vi "VariantToINIstring.vi"(7 "use system decimal point (T)":bool=TRUE, 11 "Variant-formatted Value":variant) -> (3 "String-formatted Value":string)   [LabVIEW 2013, in "OpenSerializer.lvlib" / "Serializer.PlainText.INI.lvclass"]
uses:
  Serializer.PlainText.INI.lvclass
  <vilib>/LabVIEW Open Source Project/Data Manipulation/TypeDescriptor/TypeDescriptor_GetName.vi
  <vilib>/LabVIEW Open Source Project/Data Manipulation/TypeDescriptor/TypeDescriptor_GetPString.vi
  <vilib>/LabVIEW Open Source Project/Data Manipulation/TypeDescriptor/TypeDescriptor_SetName.vi
  <vilib>/Utility/GetType.llb/Get Type Code from I16 Array And Pos.vi
  <vilib>/Utility/GetType.llb/TD_Get Array Information.vi
  <vilib>/LabVIEW Open Source Project/Data Manipulation/Conversions/Flattened nD-Array to Flattened 1D-Array.vi
  <vilib>/Utility/VariantDataType/VariantType.lvlib
  <vilib>/LabVIEW Open Source Project/Data Manipulation/Variant/OpenVariant.lvlib
  Serializer.PlainText/Serializer.PlainText.lvclass
  <vilib>/LabVIEW Open Source Project/Data Manipulation/TypeDescriptor/OpenDescriptor.lvlib
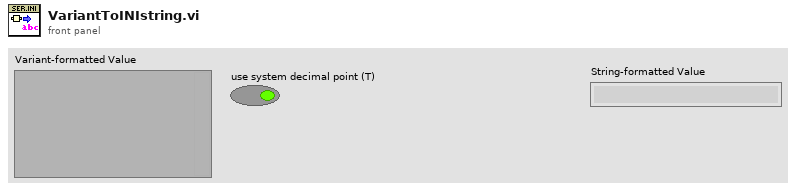
[diagram p1: front panel]
types:
  T1 = typedef "VariantType.lvlib/Type.ctl" = enum8{"Invalid Type", "Void", "I8", "I16", "I32", "I64", "U8", "U16", "U32", "U64", "Single Float", "Double Float", "Extended Float", "Single Complex", "Double Complex", "Extended Complex", "Enum U8", "Enum U16", "Enum U32", "Enum U64", "Single Float With Unit", "Double Float With Unit", "Extended Float With Unit", "Single Complex with Unit", "Double Complex with Unit", "Extended Complex with Unit", "Boolean", "String", "Path", "Picture", "Tag", "Array", "Cluster", "Variant", "LV Variant", "Waveform", "Timestamp", "Digital Waveform", "Digital Data", "ExpressData", "Refnum", "External Data", "VI", "Poly VI", "LabVIEW Class Instance", "Fixed Point"}
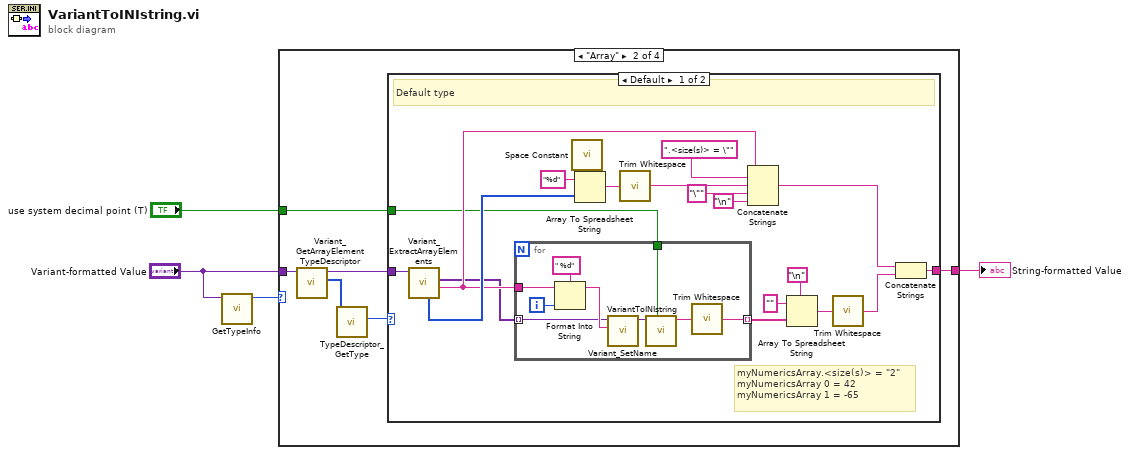
[diagram p0: block diagram]
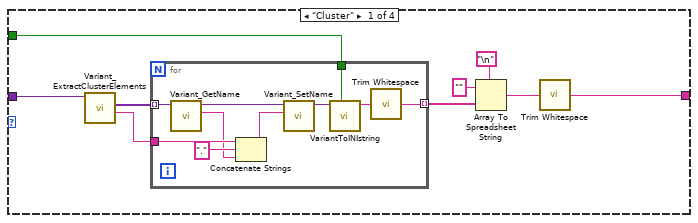
[diagram p2: hidden frame]
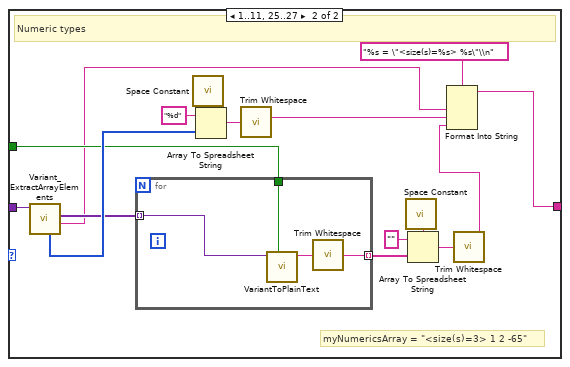
[diagram p3: hidden frame]
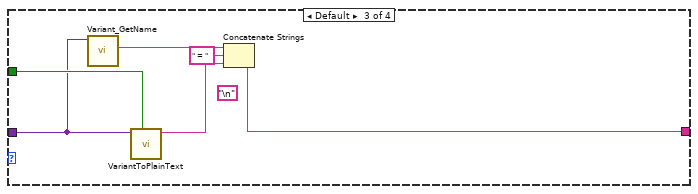
[diagram p4: hidden frame]
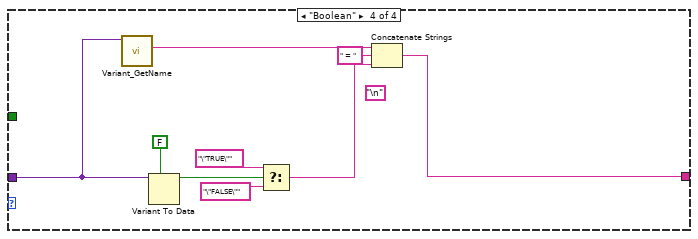
[diagram p5: hidden frame]
diagram:
  n1 = call <vilib>:"GetTypeInfo.vi"("Variant"="Variant-formatted Value") -> ("Type Enum"=w4:T1)  [unwired: 6 in, 4 out]
  n2 = case shown="\"Array\"" w4 {
    tunnel: "Variant-formatted Value" -> [w13 w26 w80 w86]
    tunnel: [w5 w29 w78 w84] -> w1
    tunnel: "use system decimal point (T)" -> [w7 w28 w83 _]
    frame "Cluster" {
      n3 = call <vilib>:"Variant_ExtractClusterElements.vi"("Cluster"=w13) -> ("name"=w9:string, "Elements"=w12:variant[])  [unwired: 8 in, 1 out]
      n4 = for {
        tunnel: w12 -> [w22] mode=indexing
        tunnel: [w14] -> w11 mode=indexing
        tunnel: w7 -> [w23]
        tunnel: w9 -> [w20]
        n5 = call <vilib>:"Variant_GetName.vi"("Variant"=w22) -> ("Name"=w19:string, "Variant dup"=w17:variant)  [unwired: 8 in, 1 out]
        n6 = Concatenate Strings(w20, "." ("string"), w19) -> (w18:string)
        n7 = call <vilib>:"Variant_SetName.vi"("Name"=w18, "Variant"=w17) -> ("Named Variant"=w16:variant)  [unwired: 9 in]
        n8 = call "VariantToINIstring.vi"("use system decimal point (T)"=w23, "Variant-formatted Value"=w16) -> ("String-formatted Value"=w15:string)  [unwired: 9 in]
        n9 = call <vilib>:"Trim Whitespace.vi"("string"=w15) -> ("trimmed string"=w14:string)  [unwired: 1 in]
      }
      n10 = Array To Spreadsheet String(delimiter (Tab)="\n", array=w11, 3:"" ("format string")) -> (spreadsheet string=w6:string)
      n11 = call <vilib>:"Trim Whitespace.vi"("string"=w6) -> ("trimmed string"=w5:string)  [unwired: 1 in]
    }
    frame "Array" {
      n12 = call <vilib>:"Variant_GetArrayElementTypeDescriptor.vi"("Array"=w26) -> ("Element Descriptor"=w27:i16[], "Array dup"=w25:variant)  [unwired: 8 in, 1 out]
      n13 = call <vilib>:"TypeDescriptor_GetType.vi"("type descriptor"=w27) -> ("Type"=w24:u8)  [unwired: 9 in, 1 out]
      n14 = case shown="Default" w24 {
        tunnel: [w48 w59] -> w29
        tunnel: w28 -> [w36 w68]
        tunnel: w25 -> [w30 w64]
        frame Default {
          # "myNumericsArray.<size(s)> = \"2\"\nmyNumericsArray 0 = 42\nmyNumericsArray 1 = -65"
          # "Default type"
          n15 = call <vilib>:"Variant_ExtractArrayElements.vi"("Array"=w30) -> ("name"=w38:string, "Elements"=w37:variant[], "Dimensions"=w44:u32[])  [unwired: 7 in, 1 out]
          n16 = for {
            tunnel: w38 -> [w53]
            tunnel: w37 -> [w49] mode=indexing
            tunnel: w36 -> [w55]
            tunnel: [w50] -> w33 mode=indexing
            i -> [w56]
            n17 = Format Into String(format string=" %d" ("Format String"), initial string=w53, w56) -> (resulting string=w52:string)  [unwired: 1 in, 1 out]
            n18 = call <vilib>:"Variant_SetName.vi"("Name"=w52, "Variant"=w49) -> ("Named Variant"=w54:variant)  [unwired: 9 in]
            n19 = call "VariantToINIstring.vi"("use system decimal point (T)"=w55, "Variant-formatted Value"=w54) -> ("String-formatted Value"=w51:string)  [unwired: 9 in]
            n20 = call <vilib>:"Trim Whitespace.vi"("string"=w51) -> ("trimmed string"=w50:string)  [unwired: 1 in]
          }
          n21 = call <vilib>:"Space Constant.vi"() -> ("String"=w47:string)
          n22 = Array To Spreadsheet String(delimiter (Tab)=w47, array=w44, 3:"%d" ("format string")) -> (spreadsheet string=w45:string)
          n23 = call <vilib>:"Trim Whitespace.vi"("string"=w45) -> ("trimmed string"=w40:string)  [unwired: 1 in]
          n24 = Concatenate Strings(w38, ".<size(s)> = \"" ("Substring"), w40, "\"" ("string"), "\n") -> (w39:string)
          n25 = Array To Spreadsheet String(delimiter (Tab)="\n", array=w33, 3:"" ("format string")) -> (spreadsheet string=w32:string)
          n26 = call <vilib>:"Trim Whitespace.vi"("string"=w32) -> ("trimmed string"=w31:string)  [unwired: 1 in]
          n27 = Concatenate Strings(w39, w31) -> (w48:string)
        }
        frame 1..11, 25..27 {
          # "myNumericsArray = \"<size(s)=3> 1 2 -65\""
          # "Numeric types"
          n28 = call <vilib>:"Variant_ExtractArrayElements.vi"("Array"=w64) -> ("name"=w63:string, "Elements"=w69:variant[], "Dimensions"=w70:u32[])  [unwired: 7 in, 1 out]
          n29 = for {
            tunnel: w69 -> [w76] mode=indexing
            tunnel: w68 -> [w75]
            tunnel: [w77] -> w66 mode=indexing
            n30 = call "VariantToPlainText.vi"("use system decimal point (T)"=w75, "Variant-formatted Value"=w76) -> ("String-formatted Value"=w74:string)  [unwired: 9 in]
            n31 = call <vilib>:"Trim Whitespace.vi"("string"=w74) -> ("trimmed string"=w77:string)  [unwired: 1 in]
          }
          n32 = call <vilib>:"Space Constant.vi"() -> ("String"=w73:string)
          n33 = Array To Spreadsheet String(delimiter (Tab)=w73, array=w70, 3:"%d" ("format string")) -> (spreadsheet string=w71:string)
          n34 = call <vilib>:"Trim Whitespace.vi"("string"=w71) -> ("trimmed string"=w61:string)  [unwired: 1 in]
          n35 = call <vilib>:"Space Constant.vi"() -> ("String"=w58:string)
          n36 = Array To Spreadsheet String(delimiter (Tab)=w58, array=w66, 3:"" ("format string")) -> (spreadsheet string=w65:string)
          n37 = call <vilib>:"Trim Whitespace.vi"("string"=w65) -> ("trimmed string"=w60:string)  [unwired: 1 in]
          n38 = Format Into String(format string="%s = \"<size(s)=%s> %s\"\\n", w63, w61, w60) -> (resulting string=w59:string)  [unwired: 2 in, 1 out]
        }
      }
    }
    frame Default {
      (unwired) "\n"
      n39 = call <vilib>:"Variant_GetName.vi"("Variant"=w80) -> ("Name"=w82:string)  [unwired: 8 in, 2 out]
      n40 = call "VariantToPlainText.vi"("use system decimal point (T)"=w83, "Variant-formatted Value"=w80) -> ("String-formatted Value"=w79:string)  [unwired: 9 in]
      n41 = Concatenate Strings(w82, " = " ("string"), w79) -> (w78:string)
    }
    frame "Boolean" {
      (unwired) "\n"
      n42 = call <vilib>:"Variant_GetName.vi"("Variant"=w86) -> ("Name"=w88:string)  [unwired: 8 in, 2 out]
      n43 = Variant To Data(type=FALSE, Variant=w86) -> (data=w91:bool)  [unwired: 1 in, 1 out]
      n44 = Select(t="\"TRUE\"", s=w91, f="\"FALSE\"") -> (s? t:f=w85:string)
      n45 = Concatenate Strings(w88, " = " ("string"), w85) -> (w84:string)
    }
  }
  "String-formatted Value" <- w1
